vi "WriteImageSize.vi"(8 "error in":errorcluster, 9 "Height":i32, 10 "Width":i32, 11 "Image Reference In":T1) -> (0 "error out":errorcluster, 3 "Image Reference Out":T1)   [LabVIEW 2020, in "OpenLvVision_Image.lvlib" / "Management.lvlib"]
doc: "Returns the image dimensions in pixel."
uses:
  Management.lvlib
  TypeDef/Image.ctl
  <vilib>/Utility/error.llb/Error Cluster From Error Code.vi
  <vilib>/ErrorRing/Error Ring.xnode
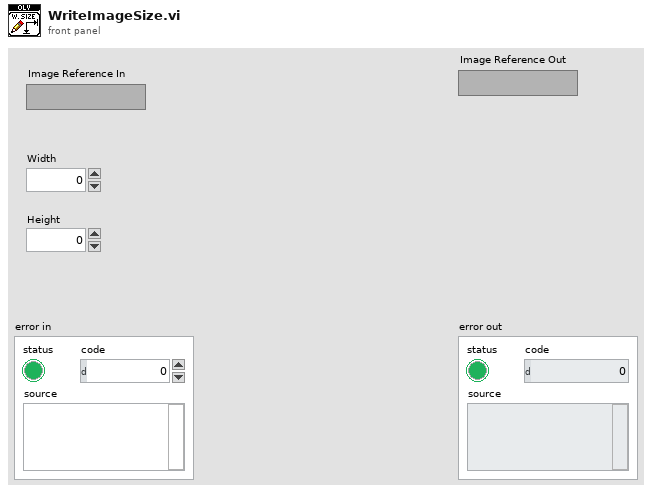
[diagram p1: front panel]
types:
  T1 = typedef "OpenLvVision_Image.lvlib/Management.lvlib/Image.ctl" = refnum<image>
  T2 = typedef "IMAQ Image.ctl" = refnum<image>
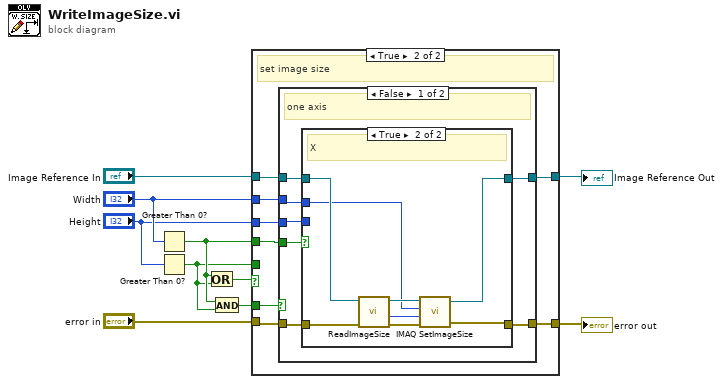
[diagram p0: block diagram]
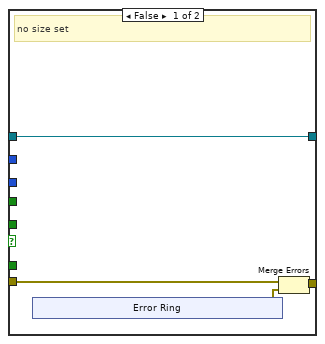
[diagram p2: hidden frame]
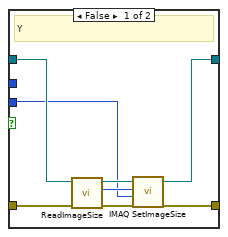
[diagram p3: hidden frame]
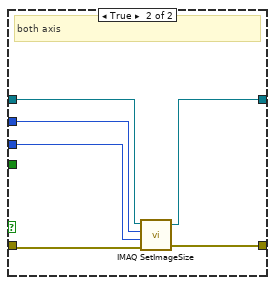
[diagram p4: hidden frame]
diagram:
  n1 = Greater Than 0?(x="Width") -> (x > 0?=w3:bool)
  n2 = Greater Than 0?(x="Height") -> (x > 0?=w2:bool)
  n3 = Or(x=w3, y=w2) -> (x .or. y?=w8:bool)
  n4 = And(x=w3, y=w2) -> (x .and. y?=w1:bool)
  n5 = case shown="True" w8 {
    tunnel: "error in" -> [w14 w26]
    tunnel: [w13 w22] -> w9
    tunnel: w3 -> [_ w19]
    tunnel: "Width" -> [_ w21]
    tunnel: "Height" -> [_ w20]
    tunnel: [w11 w23] -> w5
    tunnel: "Image Reference In" -> [w11 w24]
    tunnel: w2 -> [_ _]
    tunnel: w1 -> [_ w25]
    frame False {
      # "no size set"
      n6 = xnode "Error Ring"() -> ("error out"=w12:errorcluster)
      n7 = Merge Errors(w14, w12) -> (w13:errorcluster)
    }
    frame True {
      # "set image size"
      n8 = case shown="False" w25 {
        tunnel: w26 -> [w31 w55]
        tunnel: w24 -> [w29 w53]
        tunnel: [w30 w52] -> w23
        tunnel: [w32 w54] -> w22
        tunnel: w21 -> [w28 w51]
        tunnel: w20 -> [w27 w50]
        tunnel: w19 -> [w33 _]
        frame False {
          # "one axis"
          n9 = case shown="True" w33 {
            tunnel: [w38 w45] -> w32
            tunnel: w31 -> [w39 w49]
            tunnel: [w37 w44] -> w30
            tunnel: w29 -> [w36 w48]
            tunnel: w28 -> [_ w43]
            tunnel: w27 -> [w34 _]
            frame False {
              # "Y"
              n10 = call "ReadImageSize.vi"("error in"=w39, "Image Reference In"=w36) -> ("error out"=w41:errorcluster, "Width"=w35:i32, "Image Reference Out"=w40:T1)  [unwired: 6 in, 1 out]
              n11 = call "IMAQ SetImageSize"("error in (no error)"=w41, "Y Resolution"=w34, "X Resolution"=w35, "Image"=w40) -> ("error out"=w38:errorcluster, "Image Out"=w37:T2)  [unwired: 1 in]
            }
            frame True {
              # "X"
              n12 = call "ReadImageSize.vi"("error in"=w49, "Image Reference In"=w48) -> ("error out"=w47:errorcluster, "Height"=w42:i32, "Image Reference Out"=w46:T1)  [unwired: 6 in, 1 out]
              n13 = call "IMAQ SetImageSize"("error in (no error)"=w47, "Y Resolution"=w42, "X Resolution"=w43, "Image"=w46) -> ("error out"=w45:errorcluster, "Image Out"=w44:T2)  [unwired: 1 in]
            }
          }
        }
        frame True {
          # "both axis"
          n14 = call "IMAQ SetImageSize"("error in (no error)"=w55, "Y Resolution"=w50, "X Resolution"=w51, "Image"=w53) -> ("error out"=w54:errorcluster, "Image Out"=w52:T2)  [unwired: 1 in]
        }
      }
    }
  }
  "error out" <- w9
  "Image Reference Out" <- w5
